vi "Drive Controller.vi"(8 "error in":errorcluster) -> ()   [LabVIEW 2019]
doc: "This VI executes continuously carrying out the current operation and responding to updates or new operation requests. It will often contain the timing or control code that is difficult to place directly in TeleOp. This VI generally opens all sensors and motors and isolates the rest of the robot code from knowing implementation details of how the operations are carried out."
uses:
  <vilib>/Rock Robotics/WPI/Framework/Completion Status.ctl
  Drive Setpoints.ctl
  Drive Operations.ctl
  ADIS16470Lib/Typedef/ADIS16470 Data.ctl
  <vilib>/Rock Robotics/WPI/ThirdParty/REV Robotics/SPARK MAX/Typedef/Spark MAX Control Type.ctl
panel:
  out "ADIS16470 Value":T1
  in  "PID Constants":T2={"P Gain"=0.0005, "I Gain"=0.0, "D Gain"=0.0004, "F Gain"=0.00017, "I Zone"=0.0, "Min Output"=-1.0, "Max Output"=1.0}
  out "L setpoint":cluster{"Sensor Velocity":dbl, dbl}(graph)
  out "R setpoint":cluster{"Sensor Velocity":dbl, dbl}(graph)
  in  "Interactive Values":T3
  in  "Buttons":cluster{"Execute Cmd":bool, "Abort Cmd":bool}
  out "Command Timing":cluster{"Start Time (ms)":u32, "Iterations":i32}
  out "Status":T5
  out "Current\nCmd":string
  # "Tip: The graph shows the motor setpoints. It may also be helpful to observe inputs and sensor values.\nYou may also want to display tuning or debugging controls."
  # "Interactive Command: You may fill in the settings for a command\nand schedule it with the Execute button. You can observe and abort\nany command while fine tuning the code for the controller."
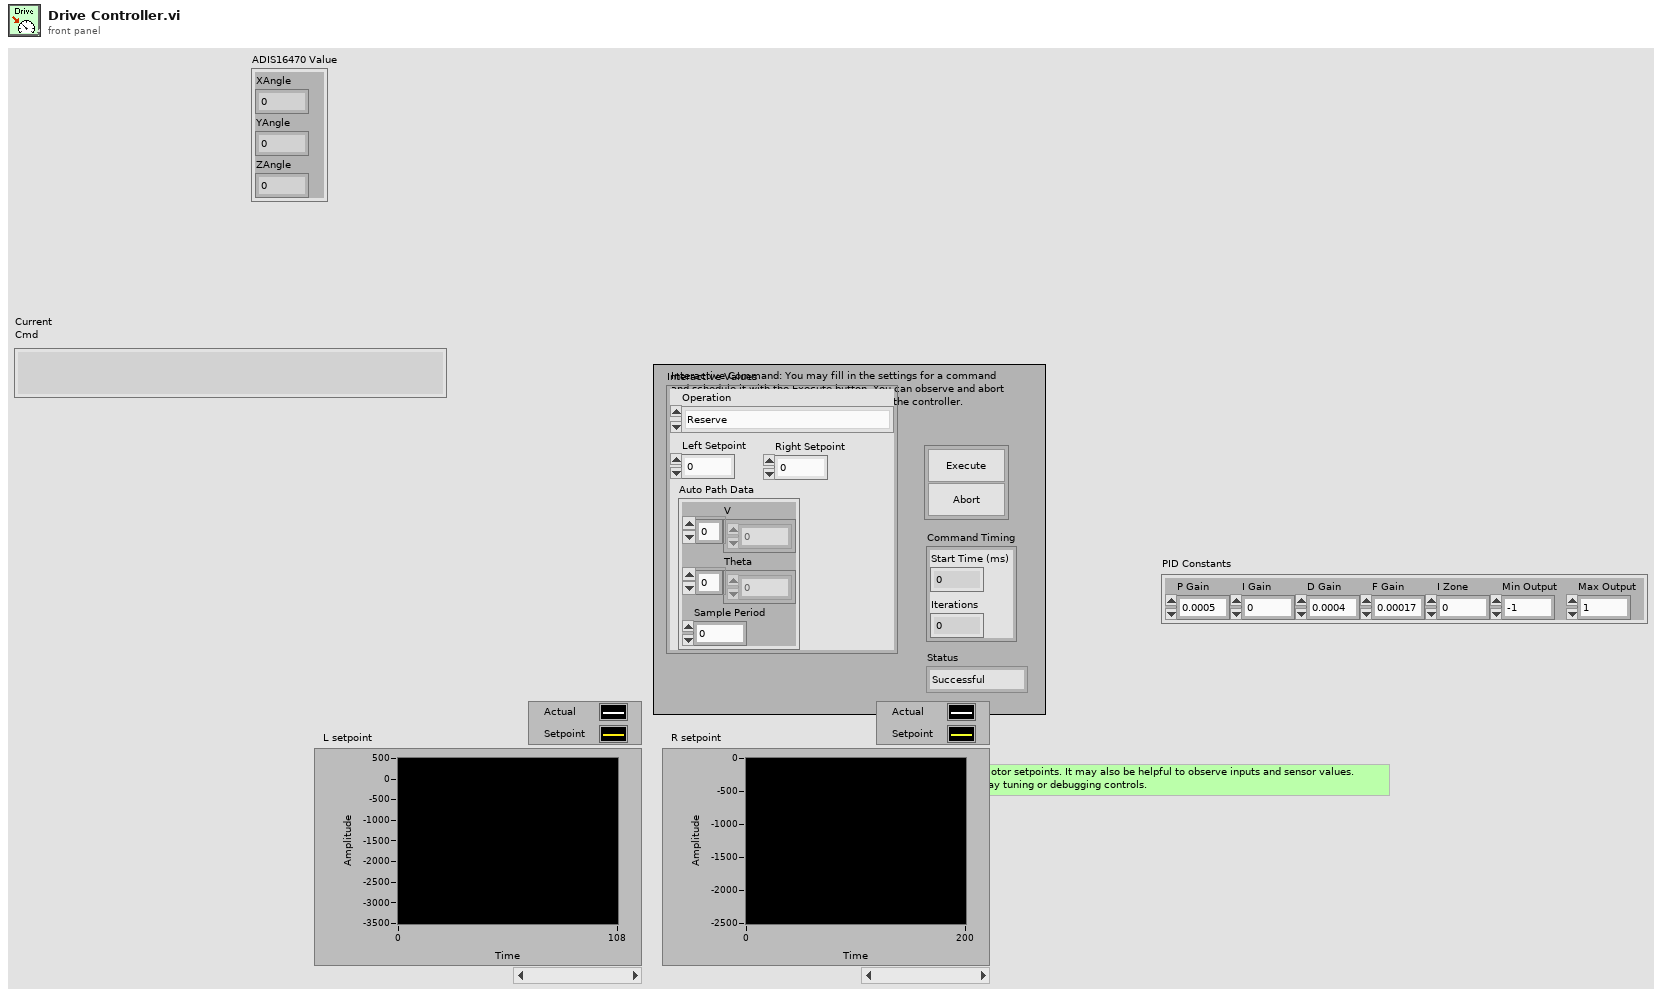
[diagram p1: front panel]
types:
  T1 = typedef "ADIS16470 Data.ctl" = cluster{"XAngle":dbl, "YAngle":dbl, "ZAngle":dbl}
  T2 = cluster{"P Gain":dbl, "I Gain":dbl, "D Gain":dbl, "F Gain":dbl, "I Zone":dbl, "Min Output":dbl, "Max Output":dbl}
  T3 = typedef "Drive Setpoints.ctl" = cluster{"Operation":T4, "Left Setpoint":dbl, "Right Setpoint":dbl, "Auto Path Data":cluster{"V":dbl[], "Theta":dbl[], "Sample Period":dbl}}
  T4 = typedef "Drive Operations.ctl" = enum16{"Reserve", "Read Current", "Immediate", "Drive for Time", "Drive for Distance", "Play Path"}
  T5 = typedef "Completion Status.ctl" = enum16{"Successful", "Aborted", "Incomplete"}
  T6 = typedef "ADIS16470 Device Reference.ctl" = cluster{"DevStatus":errorcluster, "Hardware Config":T7, "Calibration Complete":refnum<notifier>, "Status FIFO":refnum<k33>, "Last Value Reference":refnum<data-value>, "Sychronous Process VI":T11, "Cmd FIFO":refnum<k33>, "Source":T12, "Data FIFO":refnum<k33>, "Calibration Time":T16}
  T7 = typedef "ADIS16470 Hardware Configuration.ctl" = cluster{"SPI Clock Rate (Hz)":dbl, "IMU SPI Mode (3)":T8, "IMU Reset Pin":T9, "IMU SPI Bus":T10, "IMU Data Ready Pin":T9, "Stall Config":cluster{"Pow2BytesPerRead":u8, "StallTicks":u16, "CsToSclkTicks":u8}}
  T8 = typedef "WPI_SPIMode.ctl" = enum16{"Mode 0 (Clk Idle Low,Sample on Leading)", "Mode 1 (Clk Idle Low,Sample on Trailing)", "Mode 2 (Clk Idle High,Sample on Leading)", "Mode 3 (Clk Idle High,Sample on Trailing)"}
  T9 = typedef "FPGA_DIOChannel.ctl" = enum8{"DIO 0", "DIO 1", "DIO 2", "DIO 3", "DIO 4", "DIO 5", "DIO 6", "DIO 7", "DIO 8", "DIO 9", "DIO MXP 0", "DIO MXP 1", "DIO MXP 2", "DIO MXP 3", "DIO MXP 4", "DIO MXP 5", "DIO MXP 6", "DIO MXP 7", "DIO MXP 8", "DIO MXP 9", "DIO MXP 10", "DIO MXP 11", "DIO MXP 12", "DIO MXP 13", "DIO MXP 14", "DIO MXP 15", "SPI Port CS1", "SPI Port CS2", "SPI Port CS3", "SPI Port MISO", "SPI Port MOSI", "Invalid"}
  T10 = typedef "spi_bus.ctl" = enum16{"SPI On-Board, CS0", "SPI On-Board, CS1", "SPI On-Board, CS2", "SPI On-Board, CS3", "SPI MXP", "Invalid"}
  T11 = typedef "ADIS16470 Process.ctl" = refnum<vi>
  T12 = typedef "FPGA_CounterEncoderSourceConvertionLVSourceType.ctl" = cluster{"DevStatus":errorcluster, "AnalogTriggerMode?":bool, "DigitalMode":cluster{"DIO Channel":T13}, "AnalogTriggerMode":cluster{"AnalogTriggerIndex":T14, "OutputType":T15}}
  T13 = typedef "FPGA_DIODigitalSourceChannel.ctl" = enum8{"DIO 0", "DIO 1", "DIO 2", "DIO 3", "DIO 4", "DIO 5", "DIO 6", "DIO 7", "DIO 8", "DIO 9", "DIO MXP 0", "DIO MXP 1", "DIO MXP 2", "DIO MXP 3", "DIO MXP 4", "DIO MXP 5", "DIO MXP 6", "DIO MXP 7", "DIO MXP 8", "DIO MXP 9", "DIO MXP 10", "DIO MXP 11", "DIO MXP 12", "DIO MXP 13", "DIO MXP 14", "DIO MXP 15", "SPI Port CS1", "SPI Port CS2", "SPI Port CS3", "SPI Port MISO", "SPI Port MOSI", "Disabled"}
  T14 = typedef "FPGA_AnalogTriggerIndex.ctl" = enum8{"Trig 0", "Trig 1", "Trig 2", "Trig 3", "Trig 4", "Trig 5", "Trig 6", "Trig 7", "Invalid"}
  T15 = typedef "FPGA_AnalogTriggerOutType.ctl" = enum16{"InWindow", "TriggerState", "Rising", "Falling"}
  T16 = typedef "ADIS16470 Calibration Time.ctl" = enum16{"32ms", "64ms", "128ms", "256ms", "512ms", "1s", "2s", "4s", "8s", "16s", "32s", "64s"}
  T17 = typedef "WPI_MotorControlDeviceRef.ctl" = cluster{"DeviceStatus":errorcluster, "Type":T18, "PWM":cluster{"PWM Channel":T19, "DeadBand":T20}, "CAN":cluster{"Device Number":u8, "SetOutput VI Ref":variant, "GetOutput VI Ref":variant, "Enable VI Ref":variant, "Disable VI Ref":variant, "Data":variant}, "Invert":bool, "DIO PWM":cluster{"PWM \"Enable\" Channel":T19, "DIOChannel":T9, "PWM Rate":dbl}}
  T18 = typedef "WPI_MotorControlType.ctl" = enum16{"PWM", "CAN", "DIO PWM"}
  T19 = typedef "FPGA_DIOPWMChannel.ctl" = enum8{"PWM 0", "PWM 1", "PWM 2", "PWM 3", "PWM 4", "PWM 5", "PWM 6", "PWM 7", "PWM 8", "PWM 9", "PWM MXP 0", "PWM MXP 1", "PWM MXP 2", "PWM MXP 3", "PWM MXP 4", "PWM MXP 5", "PWM MXP 6", "PWM MXP 7", "PWM MXP 8", "PWM MXP 9", "Invalid"}
  T20 = typedef "WPI_PWMDeadband.ctl" = cluster{"Name":string, "maxPositivePwm":i32, "minPositivePwm":i32, "centerPwm":i32, "maxNegativePwm":i32, "minNegativePwm":i32, "angularRange":u16}
  T21 = typedef "Command Status Info.ctl" = cluster{"Name":string, "Status":T5, "notifier out":T22}
  T22 = typedef "Completion Notifier.ctl" = refnum<notifier>
  T23 = cluster{"SubSystem Data":T3, cluster{"Start Time (ms)":u32, "Iterations":i32}, cluster{"Command Info":T21, "Description":string, "Default Command":T3, "queue out":refnum<queue>, "Subsystem Name":string}}
  T24 = typedef "Spark MAX Control Type.ctl" = enum16{"Percent VBus", "Voltage", "Velocity", "Position", "Smart Motion", "Current", "Smart Velocity"}
  T25 = cluster{"V":dbl[], "Theta":dbl[], "Sample Period":dbl}
  T26 = cluster{"SubSystem Data":T3, cluster{"Start Time (ms)":u32, "Iterations":i32}, "Default Command Arguments":cluster{"Command Info":T21, "Description":string, "Default Command":T3, "queue out":refnum<queue>, "Subsystem Name":string}}
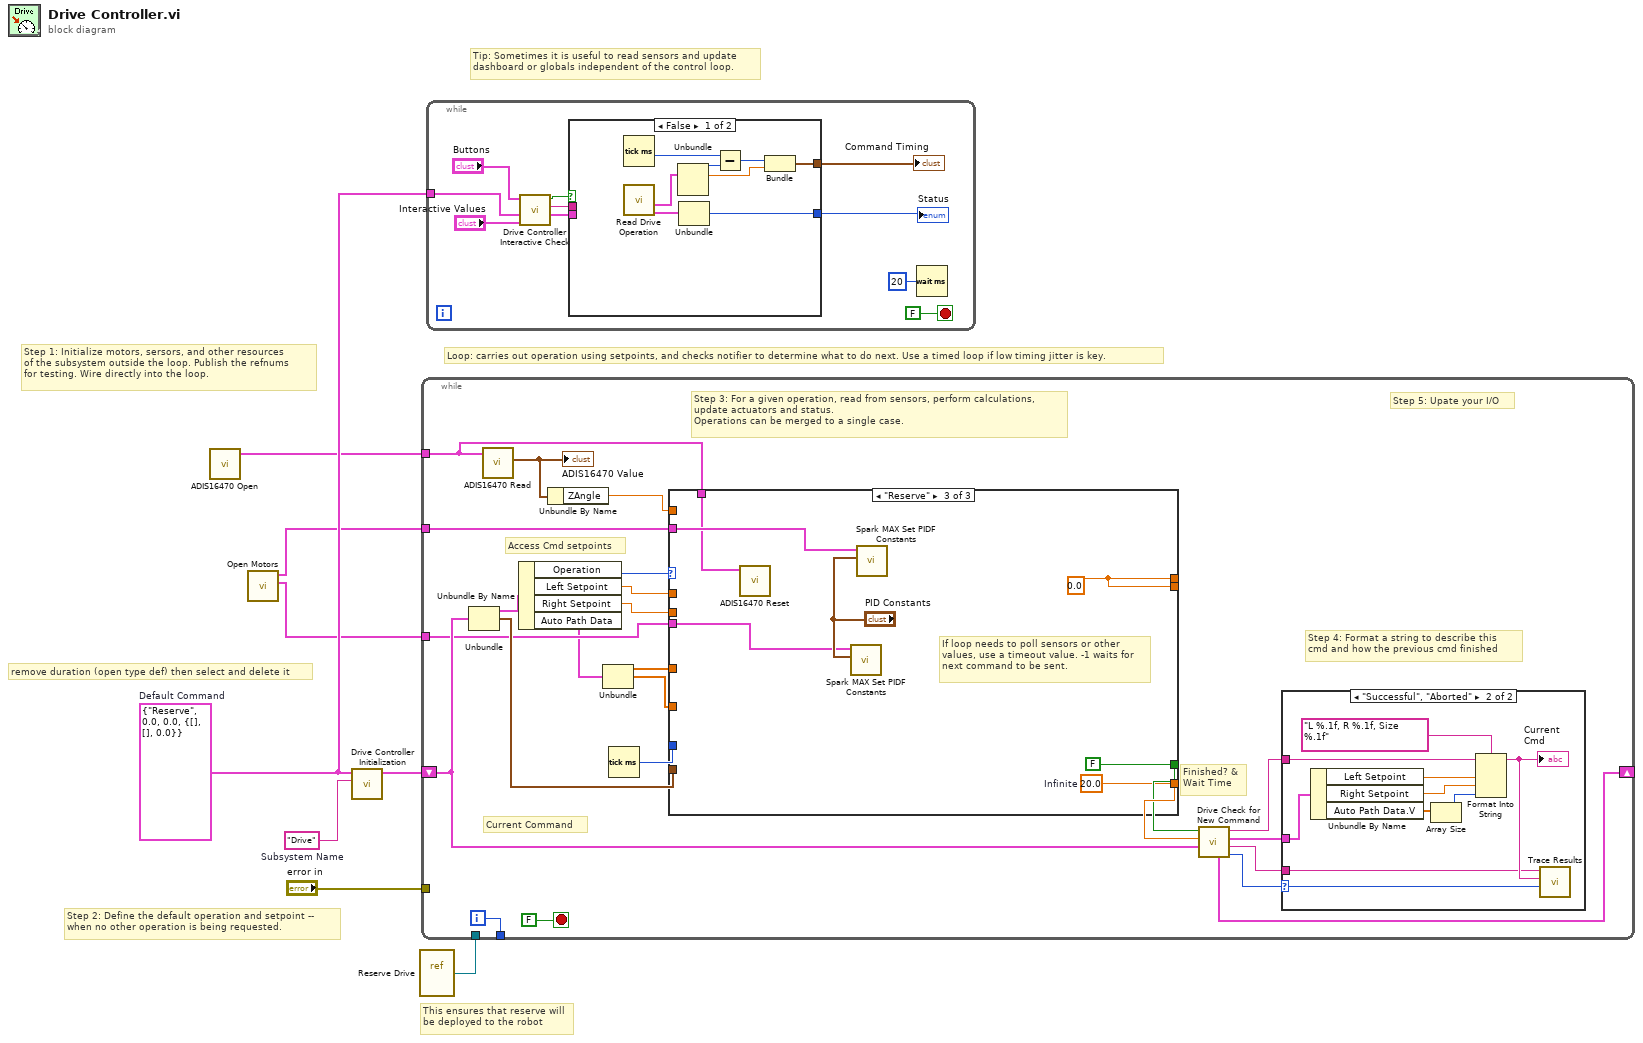
[diagram p0: block diagram]
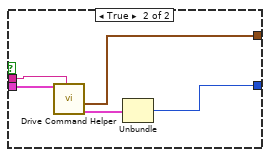
[diagram p2: hidden frame]
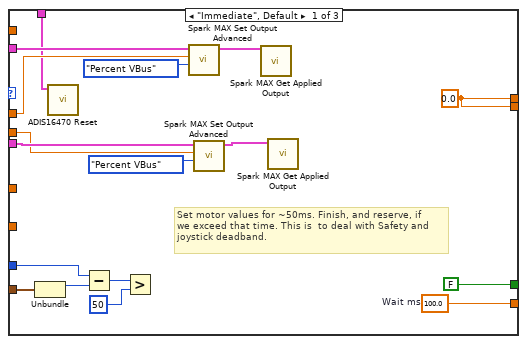
[diagram p4: hidden frame]
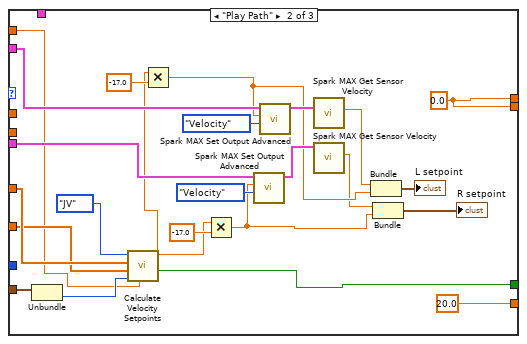
[diagram p5: hidden frame]
diagram:
  w4 = T3 {"Operation"=enum."Reserve", "Left Setpoint"=0.0, "Right Setpoint"=0.0, "Auto Path Data"={"V"=[], "Theta"=[], "Sample Period"=0.0}}  # Default Command
  w8 = "Drive"  # Subsystem Name
  # "remove duration (open type def) then select and delete it"
  # "This ensures that reserve will\nbe deployed to the robot"
  # "Tip: Sometimes it is useful to read sensors and update\ndashboard or globals independent of the control loop."
  # "Step 2: Define the default operation and setpoint --\nwhen no other operation is being requested."
  # "Step 1: Initialize motors, sersors, and other resources\nof the subsystem outside the loop. Publish the refnums\nfor testing. Wire directly into the loop."
  # "Loop: carries out operation using setpoints, and checks notifier to determine what to do next. Use a timed loop if low timing jitter is key."
  n1 = call "ADIS16470 Open.vi"() -> ("ADIS16470DevRef"=w1:T6)  [unwired: 10 in, 1 out]
  n2 = call "Open Motors.vi"() -> ("Right"=w2:T17, "Left"=w3:T17)  [unwired: 10 in]
  n3 = call "Drive Controller Initialization.vi"("Subsystem Name"=w8, "Default Command"=w4) -> ("Current Command"=w6:T23)  [unwired: 9 in]
  n4 = vi-ref "Reserve Drive.vi"() -> (w5:refnum<vi>)
  n5 = while {
    shift-right: [w25] -> _
    shift-left: w6 -> [w18]
    tunnel: [w12] -> _
    tunnel: "error in" -> [_]
    tunnel: w5 -> [_]
    tunnel: w3 -> [w17]
    tunnel: w2 -> [w16]
    tunnel: w1 -> [w9]
    i -> [w12]
    stop <- FALSE stop-if-true
    # "Step 5: Upate your I/O"
    # "Step 4: Format a string to describe this\ncmd and how the previous cmd finished"
    # "Current Command"
    # "Access Cmd setpoints"
    # "Finished? &\nWait Time"
    # "Step 3: For a given operation, read from sensors, perform calculations,\nupdate actuators and status.\nOperations can be merged to a single case."
    n6 = Unbundle(w18) -> ("SubSystem Data"=w31:T3, w19:cluster{"Start Time (ms)":u32, "Iterations":i32})  [unwired: 1 out]
    n7 = call "ADIS16470 Read.vi"("ADIS16470DevRef"=w9) -> ("ADIS16470 Value"=w11:T1)  [unwired: 7 in, 3 out]
    "ADIS16470 Value" <- w11
    n8 = Unbundle By Name(w31) -> ("Operation"=w30:T4, "Left Setpoint"=w29:dbl, "Right Setpoint"=w28:dbl, "Auto Path Data"=w15:T25)
    n9 = Unbundle By Name(w11) -> ("ZAngle"=w10:dbl)
    n10 = Unbundle(w15) -> ("V"=w14:dbl[], "Theta"=w13:dbl[])  [unwired: 1 out]
    n11 = Tick Count (ms)() -> (millisecond timer value=w27:u32)
    n12 = case shown="\"Reserve\"" w30 {
      tunnel: [w59 20.0 ("Infinite") w91] -> w24
      tunnel: [FALSE ("ignore previous (F)") w75 FALSE ("ignore previous (F)")] -> w23
      tunnel: w19 -> [w54 w62 _]
      tunnel: [w48 w84 w89] -> _
      tunnel: [w48 w84 w89] -> _
      tunnel: w29 -> [w46 _ _]
      tunnel: w28 -> [w44 _ _]
      tunnel: w27 -> [w55 _ _]
      tunnel: w17 -> [w52 w83 w87]
      tunnel: w16 -> [w49 w82 w86]
      tunnel: w14 -> [_ w77 _]
      tunnel: w13 -> [_ w76 _]
      tunnel: w10 -> [_ w60 _]
      tunnel: w9 -> [w43 _ w85]
      frame "Immediate", Default {
        w48 = 0.0
        w59 = 100.0  # Wait ms
        # "Set motor values for ~50ms. Finish, and reserve, if\nwe exceed that time. This is  to deal with Safety and\njoystick deadband."
        n13 = Unbundle(w54) -> ("Start Time (ms)"=w56:u32)  [unwired: 1 out]
        n14 = call "ADIS16470 Reset.vi"("ADIS16470DevRef"=w43) -> ()  [unwired: 9 in, 2 out]
        n15 = Subtract(x=w55, y=w56) -> (x-y=w57:u32)
        n16 = Greater?(x=w57, y=u8 50 ("Left Motor")) -> ()  [unwired: 1 out]
        n17 = call <vilib>:"Spark MAX Set Output Advanced.vi"("Control Mode"=Spark_MAX_Control_Type."Percent VBus", "Setpoint"=w46, "MotorControlDevRef"=w52) -> ("MotorControlDevRef"=w47:T17)  [unwired: 7 in, 1 out]
        n18 = call <vilib>:"Spark MAX Set Output Advanced.vi"("Control Mode"=Spark_MAX_Control_Type."Percent VBus", "Setpoint"=w44, "MotorControlDevRef"=w49) -> ("MotorControlDevRef"=w45:T17)  [unwired: 7 in, 1 out]
        n19 = call <vilib>:"Spark MAX Get Applied Output.vi"("MotorControlDevRef in"=w47) -> ()  [unwired: 7 in, 4 out]
        n20 = call <vilib>:"Spark MAX Get Applied Output.vi"("MotorControlDevRef in"=w45) -> ()  [unwired: 7 in, 4 out]
      }
      frame "Play Path" {
        w84 = 0.0
        n21 = Unbundle(w62) -> ("Iterations"=w61:i32)  [unwired: 1 out]
        n22 = call "Calculate Velocity Setpoints.vi"("IMU Input"=w60, "Iterations"=w61, "Angular Data (Relative)"=w76, "Velocity Data"=w77, "Enum"=enum16{"JV", "Mule", "Linda/Sophie"}."JV") -> ("Finished?"=w75:bool, "Right Setpoint"=w71:dbl, "Left Setpoint"=w72:dbl)  [unwired: 4 in]
        n23 = Multiply(x=w71, y=-17.0) -> (x*y=w68:dbl)
        n24 = Multiply(x=w72, y=-17.0) -> (x*y=w64:dbl)
        n25 = call <vilib>:"Spark MAX Set Output Advanced.vi"("Control Mode"=Spark_MAX_Control_Type."Velocity", "Setpoint"=w64, "MotorControlDevRef"=w82) -> ("MotorControlDevRef"=w69:T17)  [unwired: 7 in, 1 out]
        n26 = call <vilib>:"Spark MAX Set Output Advanced.vi"("Control Mode"=Spark_MAX_Control_Type."Velocity", "Setpoint"=w68, "MotorControlDevRef"=w83) -> ("MotorControlDevRef"=w70:T17)  [unwired: 7 in, 1 out]
        n27 = call <vilib>:"Spark MAX Get Sensor Velocity.vi"("MotorControlDevRef in"=w70) -> ("Sensor Velocity"=w67:dbl)  [unwired: 7 in, 3 out]
        n28 = call <vilib>:"Spark MAX Get Sensor Velocity.vi"("MotorControlDevRef in"=w69) -> ("Sensor Velocity"=w65:dbl)  [unwired: 7 in, 3 out]
        n29 = Bundle("Sensor Velocity"=w67, w68) -> (→"L setpoint":cluster{"Sensor Velocity":dbl, dbl})  [unwired: 1 in]
        n30 = Bundle("Sensor Velocity"=w65, w64) -> (→"R setpoint":cluster{"Sensor Velocity":dbl, dbl})  [unwired: 1 in]
      }
      frame "Reserve" {
        w89 = 0.0
        w91 = 20.0  # Infinite
        # "If loop needs to poll sensors or other\nvalues, use a timeout value. -1 waits for\nnext command to be sent."
        n31 = call "ADIS16470 Reset.vi"("ADIS16470DevRef"=w85) -> ()  [unwired: 9 in, 2 out]
        n32 = call <vilib>:"Spark MAX Set PIDF Constants.vi"("PID Constants"="PID Constants", "MotorControlDeviceRef"=w86) -> ()  [unwired: 8 in, 2 out]
        n33 = call <vilib>:"Spark MAX Set PIDF Constants.vi"("PID Constants"="PID Constants", "MotorControlDeviceRef"=w87) -> ()  [unwired: 8 in, 2 out]
      }
    }
    n34 = call "Drive Check for New Command.vi"("input cluster"=w18, "Wait time (ms)"=w24, "Finished?"=w23) -> ("Completion"=w26:T5, "Subsystem Name"=w20:string, "Current Command"=w21:T3, "Initial Trace String"=w22:string, "Next Command"=w25:T26)  [unwired: 4 in]
    n35 = case shown="\"Successful\", \"Aborted\"" w26 {
      selector: w26 -> [_ w42]
      tunnel: w22 -> [_ w37]
      tunnel: w21 -> [_ w38]
      tunnel: w20 -> [_ w35]
      frame "Incomplete", Default {
        # "Continuing current command"
      }
      frame "Successful", "Aborted" {
        # "Report and setup for next command"
        n36 = Unbundle By Name(w38) -> ("Left Setpoint"=w40:dbl, "Right Setpoint"=w41:dbl, "Auto Path Data.V"=w34:dbl[])
        n37 = Array Size(array=w34) -> (size(s)=w33:i32)
        n38 = Format Into String(format string="L %.1f, R %.1f, Size %.1f", initial string=w37, w40, w41, w33) -> (resulting string=w36:string)  [unwired: 1 in, 1 out]
        "Current\nCmd" <- w36
        n39 = call <vilib>:"Trace Results.vi"("Status of previous command"=w42, "Description"=w36, "Subsystem"=w35) -> ()  [unwired: 9 in]
      }
    }
  }
  n40 = while {
    tunnel: w4 -> [w93]
    stop <- FALSE stop-if-true
    n41 = call "Drive Controller Interactive Check.vi"("Interactive Command In"="Interactive Values", "Default Command"=w93, "Buttons"="Buttons") -> ("Interactive Command Out"=w95:T3, "Trace String"=w96:string, "Schedule"=w97:bool)  [unwired: 6 in]
    n42 = case shown="False" w97 {
      tunnel: [w106 w114] -> w98
      tunnel: [w105 w110] -> w99
      tunnel: w96 -> [_ w112]
      tunnel: w95 -> [_ w111]
      frame False {
        n43 = Tick Count (ms)() -> (millisecond timer value=w109:u32)
        n44 = call "Read Drive Operation.vi"() -> ("Command Info"=w103:T21, "SubSystem Data"=w102:T3)  [unwired: 9 in, 1 out]
        n45 = Unbundle(w102) -> ("Operation"=w107:T4, "Left Setpoint"=w104:dbl)  [unwired: 2 out]
        n46 = Unbundle(w103) -> ("Status"=w106:T5)  [unwired: 2 out]
        n47 = Subtract(x=w109, y=w107) -> (x-y=w108:u32)
        n48 = Bundle(w108, "Left Setpoint"=w104) -> (w105:cluster{u32, "Left Setpoint":dbl})  [unwired: 1 in]
      }
      frame True {
        n49 = call "Drive Command Helper.vi"("Description"=w112, "SubSystem Data"=w111) -> ("Command Info Out"=w113:T21, "Command Timing"=w110:cluster{"Start Time (ms)":u32, "Iterations":i32})  [unwired: 7 in, 1 out]
        n50 = Unbundle(w113) -> ("Status"=w114:T5)  [unwired: 2 out]
      }
    }
    "Status" <- w98
    "Command Timing" <- w99
    n51 = Wait (ms)(milliseconds to wait=u32 20) -> ()  [unwired: 1 out]
  }
